vi "Remove N Packages from Feed.vi"(8 "error in":errorcluster, 9 "delete package files? (F)":bool, 10 "package filenames":string[](array[string]), 11 "feed folderpath in":path) -> (0 "error out":errorcluster, 1 "package filepaths deleted":path[](array[path]), 2 "package filenames removed from feed":string[](array[string]), 3 "feed folderpath out":path)   [LabVIEW 2014, in "NIPM_API.lvlib"]
doc: "Removes multiple packages from a feed\n\nINPUT(s)\n<B>Feed folderpath</B>: Specifies the folder containing the feed\n\n<B>Package filenames</B>: Specifies the filenames of multiple packages to be removed from the feed\n\n<B>Delete package files?</B>: If this input is set to TRUE, this VI will delete the package files (.nipkg) in the feed folderpath after removing the packages from the feed. If this input is set to FALSE, the package files (.nipkg) will remain in the feed folderpath after removing the packages from the feed.\n\nOUTPUT(s)\n<B>Feed folderpath out</B>: Outputs the specified feed folderpath\n\n<B>Package filenames removed from feed</B>: Outputs the filenames of the packages that were removed from the feed\n\n<B>Package filepaths deleted</B>: Outputs the filepaths of the packages that were deleted from the feed folderpath\n\nDETAILS\nIf you specify a package filename that does not exist in the specified feed, this VI will not try to remove the package from the feed or delete the corresponding package file (.nipkg)."
uses:
  NIPM_API.lvlib
  _support/Version Comparison Operator.ctl
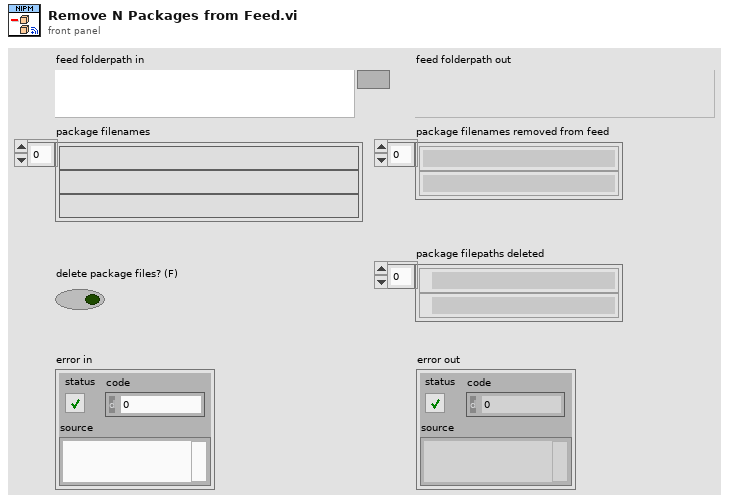
[diagram p1: front panel]
types:
  T1 = typedef "NIPM_API.lvlib/Version Comparison Operator.ctl" = enum16{">", ">=", "=", "!=", "<=", "<"}
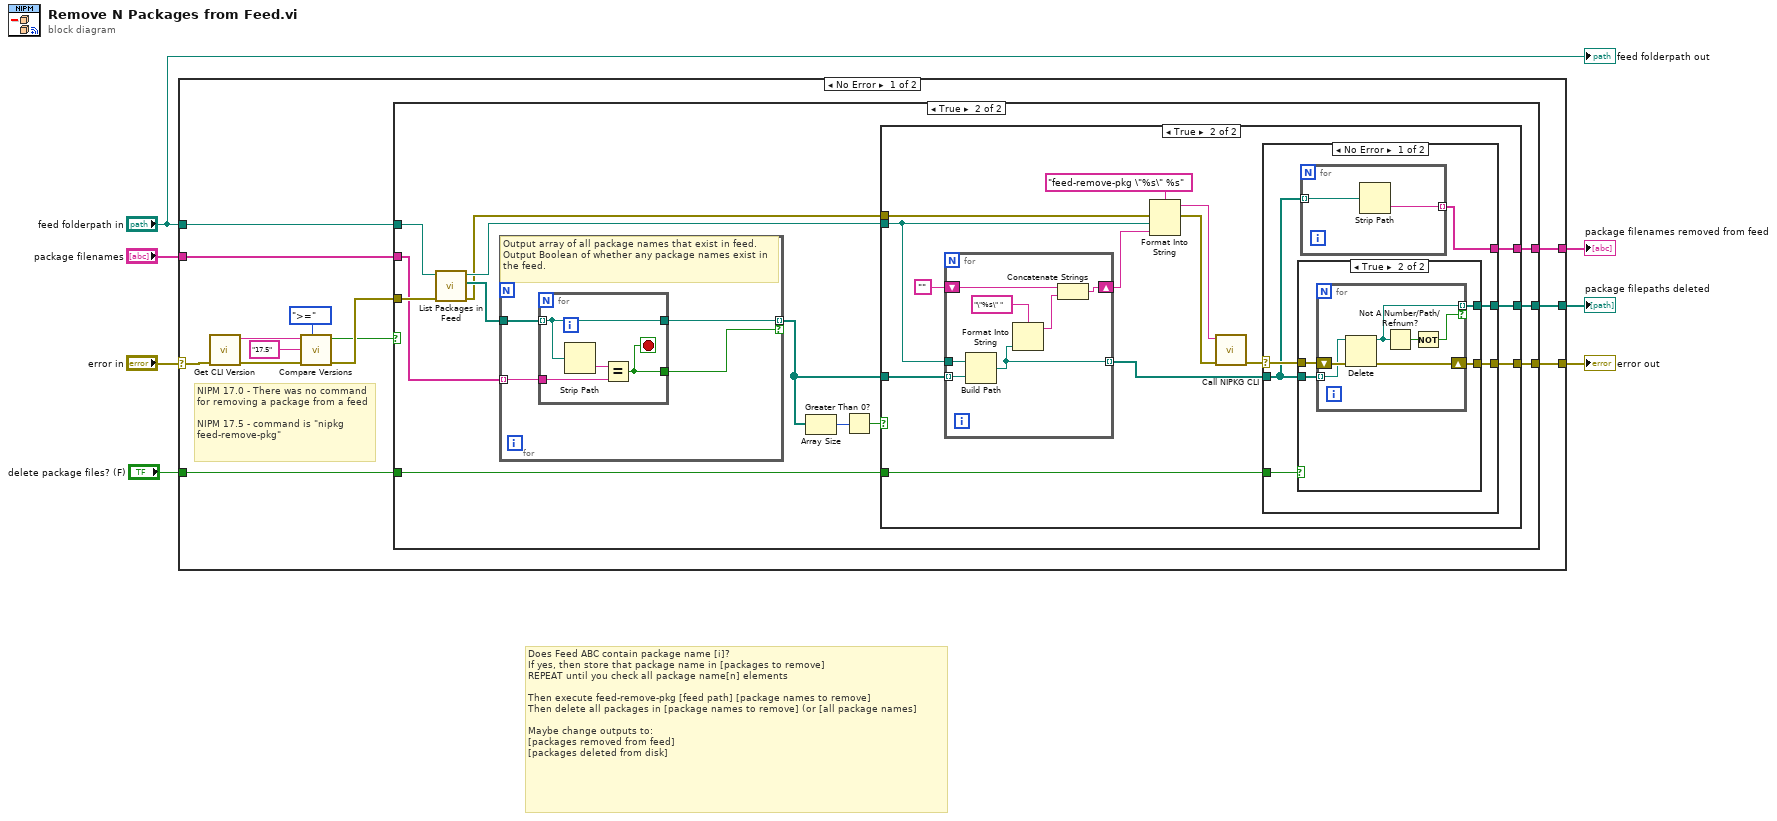
[diagram p0: block diagram]
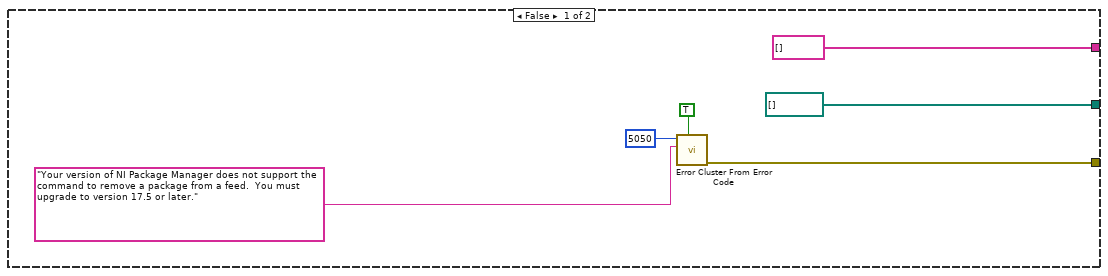
[diagram p2: hidden frame]
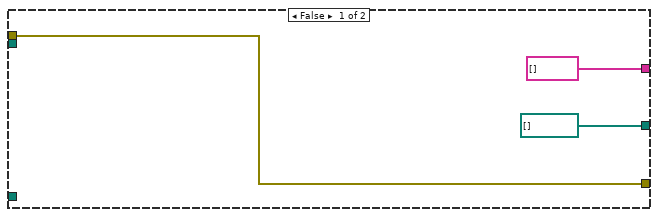
[diagram p3: hidden frame]
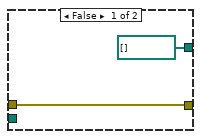
[diagram p4: hidden frame]
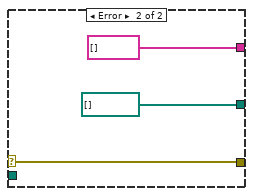
[diagram p5: hidden frame]
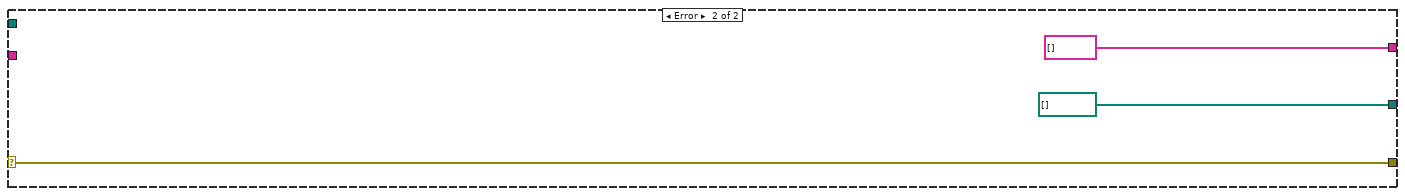
[diagram p6: hidden frame]
diagram:
  # "Does Feed ABC contain package name [i]?\nIf yes, then store that package name in [packages to remove]\nREPEAT until you check all package name[n] elements\n\nThen execute feed-remove-pkg [feed path] [package names to remove]\nThen delete all packages in [package names to remove] (or [all package names]\n\nMaybe change outputs to:\n[packages removed from feed]\n[packages deleted from disk]"
  n1 = case shown="No Error" "error in" {
    selector: "error in" -> [w17 w97]
    tunnel: [w20 w97] -> w7
    tunnel: "feed folderpath in" -> [w19 _]
    tunnel: "package filenames" -> [w18 _]
    tunnel: [w10 string[] []] -> w2
    tunnel: "delete package files? (F)" -> [w9 _]
    tunnel: [w8 path[] []] -> w1
    frame No Error {
      # "NIPM 17.0 - There was no command for removing a package from a feed\n\nNIPM 17.5 - command is \"nipkg feed-remove-pkg\""
      n2 = call "Get CLI Version.vi"("error in"=w17) -> ("error out"=w13:errorcluster, "full version string"=w14:string)  [unwired: 9 in]
      n3 = call "Compare Versions.vi"("operator"=Version_Comparison_Operator.">=", "error in"=w13, "version y"="17.5", "version x"=w14) -> ("error out"=w12:errorcluster, "Satisfied?"=w11:bool)  [unwired: 6 in]
      n4 = case shown="True" w11 {
        tunnel: [w23 w38] -> w20
        tunnel: w19 -> [_ w35]
        tunnel: w18 -> [_ w32]
        tunnel: w12 -> [_ w36]
        tunnel: [string[] [] w37] -> w10
        tunnel: w9 -> [_ w39]
        tunnel: [path[] [] w27] -> w8
        frame False {
          n5 = call <vilib>:"Error Cluster From Error Code.vi"("show call chain? (False)"=TRUE, "error message (\"\")"="Your version of NI Package Manager does not support the command to remove a package from a feed.  You must upgrade to version 17.5 or later.", "error code (0)"=5050) -> ("error out"=w23:errorcluster)  [unwired: 6 in]
        }
        frame True {
          n6 = call "List Packages in Feed.vi"("error in"=w36, "feed folderpath in"=w35) -> ("error out"=w31:errorcluster, "package relative filepaths"=w33:path[], "feed folderpath out"=w34:path)  [unwired: 6 in, 1 out]
          n7 = for {
            tunnel: w33 -> [w90]
            tunnel: w32 -> [w89] mode=indexing
            tunnel: [w88] -> w29 mode=indexing if=w87
            # "Output array of all package names that exist in feed.\nOutput Boolean of whether any package names exist in the feed."
            n8 = for {
              tunnel: w90 -> [w91] mode=indexing
              tunnel: w89 -> [w93]
              tunnel: [w92] -> w87
              tunnel: [w91] -> w88
              stop <- w92 stop-if-true
              n9 = Strip Path(path=w91) -> (name=w94:string)  [unwired: 1 out]
              n10 = Equal?(x=w94, y=w93) -> (x = y?=w92:bool)
            }
          }
          n11 = Array Size(array=w29) -> (size(s)=w28:i32)
          n12 = Greater Than 0?(x=w28) -> (x > 0?=w30:bool)
          n13 = case shown="True" w30 {
            tunnel: w39 -> [_ w53]
            tunnel: [w42 w51] -> w38
            tunnel: [string[] [] w43] -> w37
            tunnel: w34 -> [_ w49]
            tunnel: w29 -> [_ w48]
            tunnel: w31 -> [w42 w50]
            tunnel: [path[] [] w45] -> w27
            frame False {
            }
            frame True {
              n14 = for {
                tunnel: w48 -> [w85] mode=indexing
                tunnel: w49 -> [w86]
                tunnel: [w83] -> w44 mode=indexing
                shift-right: [w82] -> w46
                shift-left: "" -> [w81]
                n15 = Build Path(base path=w86, name or relative path=w85) -> (appended path=w83:path)
                n16 = Format Into String(format string="\"%s\" ", w83) -> (resulting string=w80:string)  [unwired: 2 in, 1 out]
                n17 = Concatenate Strings(w81, w80) -> (w82:string)
              }
              n18 = Format Into String(format string="feed-remove-pkg \"%s\" %s", error in=w50, w49, w46) -> (resulting string=w55:string, error out=w54:errorcluster)  [unwired: 1 in]
              n19 = call "Call NIPKG CLI.vi"("error in (no error)"=w54, "command"=w55) -> ("error out"=w52:errorcluster)  [unwired: 8 in, 1 out]
              n20 = case shown="No Error" w52 {
                selector: w52 -> [w61 w77]
                tunnel: w53 -> [w62 _]
                tunnel: [w60 w77] -> w51
                tunnel: [w59 path[] []] -> w45
                tunnel: w44 -> [w58 _]
                tunnel: [w57 string[] []] -> w43
                frame No Error {
                  n21 = case shown="True" w62 {
                    tunnel: w61 -> [w66 w70]
                    tunnel: [w66 w69] -> w60
                    tunnel: w58 -> [_ w68]
                    tunnel: [path[] [] w67] -> w59
                    frame False {
                    }
                    frame True {
                      n22 = for {
                        tunnel: w68 -> [w73] mode=indexing
                        shift-right: [w75] -> w69
                        shift-left: w70 -> [w76]
                        tunnel: [w72] -> w67 mode=indexing if=w71
                        n23 = Delete(path (use dialog)=w73, error in=w76) -> (deleted path=w72:path, error out=w75:errorcluster)  [unwired: 3 in, 1 out]
                        n24 = Not A Number/Path/Refnum?(number/path/refnum=w72) -> (NaN/Path/Refnum?=w74:bool)
                        n25 = Not(x=w74) -> (.not. x?=w71:bool)
                      }
                    }
                  }
                  n26 = for {
                    tunnel: w58 -> [w64] mode=indexing
                    tunnel: [w63] -> w57 mode=indexing
                    n27 = Strip Path(path=w64) -> (name=w63:string)  [unwired: 1 out]
                  }
                }
                frame Error {
                }
              }
            }
          }
        }
      }
    }
    frame Error {
    }
  }
  "error out" <- w7
  "package filenames removed from feed" <- w2
  "package filepaths deleted" <- w1
  "feed folderpath out" <- "feed folderpath in"
